vi "Pre Launch Init.vi"(11 "Nested in":refnum<class "Database Provider.lvclass">) -> (0 "error out":errorcluster, 3 "Nested out":refnum<class "Database Provider.lvclass">)   [LabVIEW 2023, in "Database Provider.lvlib" / "Database Provider.lvclass"]
doc: "(<B>Filename</B>: Actor Framework.lvlib:Actor.lvclass:Pre Launch Init.vi)\n\nDefines behavior that occurs after the Launch Nested Actor method is invoked but before the actor's Actor Core method begins running.\n\nBy default, this method does nothing. A descendant class may override it to define behavior."
uses:
  Database Provider.lvclass
  Database Provider.lvclass/Database Provider.ctl
  <vilib>/MGI/Panel Manager/Panel Actor/Panel Actor/Panel Actor.lvclass
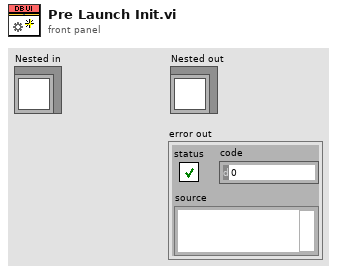
[diagram p1: front panel]
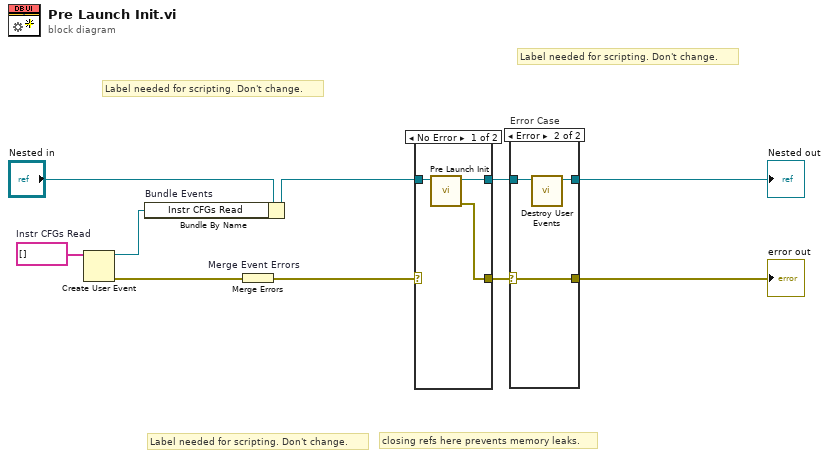
[diagram p0: block diagram]
diagram:
  w2 = string[] []  # Instr CFGs Read
  # "Label needed for scripting. Don't change."
  # "Label needed for scripting. Don't change."
  # "Label needed for scripting. Don't change."
  # "closing refs here prevents memory leaks."
  n1 = Create User Event(user event datatype=w2) -> (user event=w1:refnum<user-event>, error out=w9:errorcluster)  [unwired: 1 in]
  n2 = Bundle By Name "Bundle Events"(cluster="Nested in", "Instr CFGs Read"=w1) -> (w5:refnum<class "Database Provider.lvclass">)
  n3 = Merge Errors "Merge Event Errors"(w9) -> (w4:errorcluster)
  n4 = case shown="No Error" w4 {
    selector: w4 -> [_ w15]
    tunnel: [w13 w14] -> w6
    tunnel: w5 -> [w12 w14]
    tunnel: [w11 w15] -> w3
    frame No Error {
      n5 = call-parent "Pre Launch Init.vi"("Panel Actor in"=w12) -> ("error out"=w11:errorcluster, "Panel Actor out"=w13:refnum<class "Database Provider.lvclass">)  [unwired: 9 in]
    }
    frame Error {
    }
  }
  n6 = case "Error Case" shown="Error" w3 {
    selector: w3 -> [w16 w20]
    tunnel: w6 -> [w17 w19]
    tunnel: [w17 w18] -> w8
    tunnel: [w16 w20] -> w7
    frame No Error {
    }
    frame Error {
      n7 = call "Destroy User Events.vi"("UI Template in"=w19) -> ("UI Template out"=w18:refnum<class "Database Provider.lvclass">)  [unwired: 10 in]
    }
  }
  "error out" <- w7
  "Nested out" <- w8
